vi "appendTable--double.vi"(8 "error in (no error)":errorcluster, 9 "Font":refnum<class "Style.lvclass">, 10 "Table":dbl[][](array[numeric]), 11 "MS-Word in":refnum<class "MS-Word.lvclass">) -> (0 "error out":errorcluster, 3 "MS-Word out":refnum<class "MS-Word.lvclass">)   [LabVIEW 2017, in "LabVIEW NPOI.lvlib" / "MS-Word.lvclass"]
doc: "Protected dynamic dispatch method to append the wire <b>Table</b> as 2D array of doubles to the <b>Document</b> as a table."
uses:
  MS-Word.lvclass
  Styles/Style/Style.lvclass
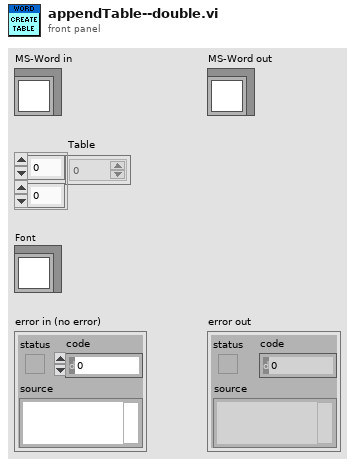
[diagram p1: front panel]
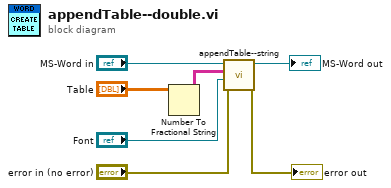
[diagram p0: block diagram]
diagram:
  n1 = Number To Fractional String(number="Table") -> (F-format string=w4:string[][])  [unwired: 3 in]
  n2 = call-dynamic "appendTable--string.vi"("error in (no error)"="error in (no error)", "Font"="Font", "Table"=w4, "MS-Word in"="MS-Word in") -> ("error out"=→"error out":errorcluster, "MS-Word out"=→"MS-Word out":refnum<class "MS-Word.lvclass">)  [unwired: 6 in]
